vi "H5Lget_val_by_idx.vi"   [LabVIEW 2017]
doc: "Retrieves value of the nth link in a group, according to the order within an index."
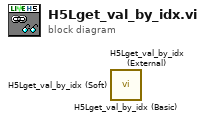
[diagram p0: block diagram]
diagram:
  n1 = call <vilib>:"H5Lget_val_by_idx (Basic).vi"() -> ()  [unwired: 8 in, 4 out]
  n2 = call <vilib>:"H5Lget_val_by_idx (External).vi"() -> ()  [unwired: 7 in, 5 out]
  n3 = call <vilib>:"H5Lget_val_by_idx (Soft).vi"() -> ()  [unwired: 8 in, 4 out]
